vi "Stop Core.vi"(10 "final error code":i32, 11 "WebSocket Client in":refnum<class "WebSocket Client.lvclass">) -> (3 "WebSocket Client out":refnum<class "WebSocket Client.lvclass">)   [LabVIEW 2017, in "WebSocket Client.lvlib" / "WebSocket Client.lvclass"]
doc: "(<B>Filename</B>: Actor Framework.lvlib:Actor.lvclass:Stop Core.vi)\n\nDefines what the actor does before it stops. Use the <B>final error code</B> input to determine whether the actor shut down in response to an error.\n\nBy default, this method does nothing. A descendant class may override it to define behavior, such as shutting down any processes the actor initiated in its override of the Actor Core method."
uses:
  WebSocket Client.lvclass
  Applications/National Instruments/LabVIEW 2017 64-bit/vi.lib/ActorFramework/Actor/Actor.lvclass
  <vilib>/ActorFramework/Actor/Actor.lvclass/Actor.ctl
  WebSocket Client.lvclass/WebSocket Client.ctl
  <vilib>/ActorFramework/Message Enqueuer/Message Enqueuer.lvclass/Message Enqueuer.ctl
  <vilib>/ActorFramework/Message Enqueuer/Enqueue.vi
  <vilib>/ActorFramework/Stop Msg/Stop Msg.lvclass
  Applications/National Instruments/LabVIEW 2017 64-bit/vi.lib/ActorFramework/Message/Message.lvclass
  <vilib>/ActorFramework/Message Priority Queue/Priority Enqueue.vi
  Actor wHelper/Actor wHelper/Actor wHelper.lvclass
  <vilib>/MediaMongrels Ltd/WebSockets/Sockets/VISA TCP Socket/VISA TCP.lvclass
  <vilib>/ActorFramework/Actor/Actor.lvclass
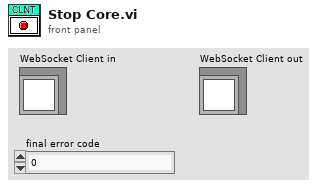
[diagram p1: front panel]
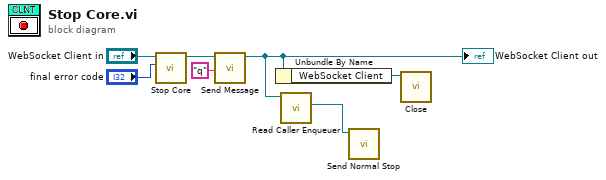
[diagram p0: block diagram]
diagram:
  n1 = call-parent "Stop Core.vi"("final error code"="final error code", "Actor wHelper in"="WebSocket Client in") -> ("Actor wHelper out"=w4:refnum<class "WebSocket Client.lvclass">)  [unwired: 9 in]
  n2 = call "Send Message.vi"("Message"="q", "WebSocket Client in"=w4) -> ("WebSocket Client out"=w2:refnum<class "WebSocket Client.lvclass">)  [unwired: 8 in, 1 out]
  "WebSocket Client out" <- w2
  n3 = Unbundle By Name(w2) -> ("WebSocket Client"=w5:refnum<class "VISA TCP.lvclass">)
  n4 = call <vilib>:"Read Caller Enqueuer.vi"("Actor"=w2) -> ("Caller Enqueuer"=w1:refnum<class "Message Enqueuer.lvclass">)  [unwired: 10 in]
  n5 = call <vilib>:"Send Normal Stop.vi"("Message Enqueuer"=w1) -> ()  [unwired: 10 in, 1 out]
  n6 = call-dynamic "Close.vi"("VISA TCP in"=w5) -> ()  [unwired: 10 in, 1 out]
